vi "algorithm.vi"(1 "x":dbl) -> (0 "f(x)":dbl)   [LabVIEW 2011]
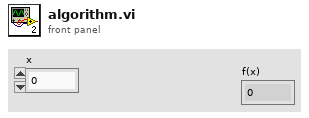
[diagram p1: front panel]
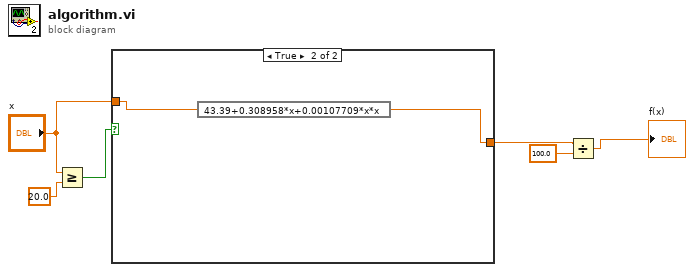
[diagram p0: block diagram]
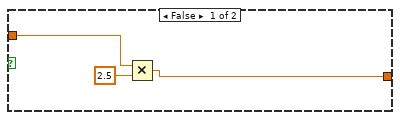
[diagram p2: hidden frame]
diagram:
  n1 = Greater Or Equal?(x="x", y=20.0) -> (x >= y?=w4:bool)
  n2 = case shown="True" w4 {
    tunnel: "x" -> [w8 w11]
    tunnel: [w7 w10] -> w3
    frame False {
      n3 = Multiply(x=w8, y=2.5) -> (x*y=w7:dbl)
    }
    frame True {
      n4 = expression code="43.39+0.308958*x+0.00107709*x*x"(w11) -> (w10:dbl)
    }
  }
  n5 = Divide(x=w3, y=100.0) -> (x/y=→"f(x)":dbl)
